vi "ID Pool.Return ID to Pool.vi"(8 "error in (no error)":errorcluster, 9 "timeout in ms (0)":i32 format="%d ms", 10 "id":i32, 11 "ID Pool in":refnum<class "ID Pool.lvclass">) -> (0 "error out":errorcluster, 1 "timed out?":bool, 3 "ID Pool out":refnum<class "ID Pool.lvclass">)   [LabVIEW 2017, in "DSF.Engine.lvlib" / "ID Pool.lvclass"]
uses:
  ID Pool.lvclass
  C:/Git/DSF/dsf core/Source/Engine/Classes/Thread Pool/Pool.lvclass
  Pool.lvclass/Pool.ctl
  Debug/DSF.Engine.Debug Flags.FIFO.lvclass/DSF.Engine.Debug Flags.FIFO.ctl
  Pool.Get FIFO.vi
  Pool.Get Debug Flags.vi
  Debug/DSF.Engine.Debug Flags.FIFO.Get Infinite Timeouts.vi
  Pool.lvclass
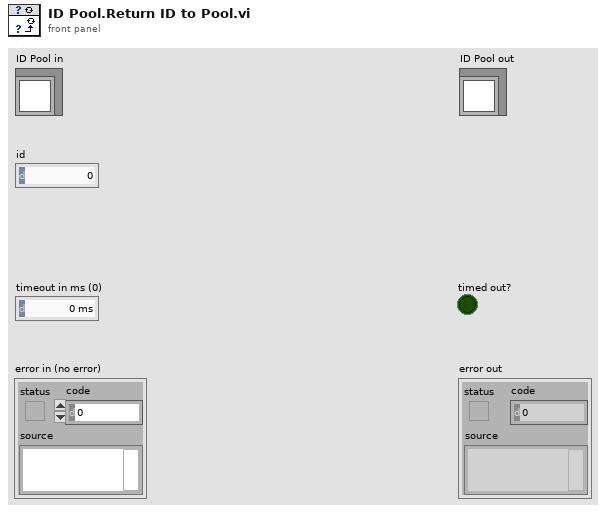
[diagram p1: front panel]
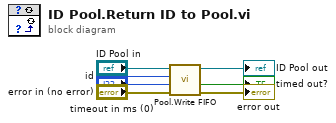
[diagram p0: block diagram]
diagram:
  n1 = call "Pool.Write FIFO.vi"("error in (no error)"="error in (no error)", "timeout in ms (0)"="timeout in ms (0)", "element"="id", "Pool in"="ID Pool in") -> ("error out"=→"error out":errorcluster, "timed out?"=→"timed out?":bool, "Pool out"=→"ID Pool out":refnum<class "ID Pool.lvclass">)  [unwired: 5 in]
